vi "DAC Configure FP View.vi"(8 "error in":errorcluster, 11 "DAC RTD Temp in":refnum<class "DAC RTD Temp.lvclass">) -> (0 "error out":errorcluster, 3 "DAC RTD Temp out":refnum<class "DAC RTD Temp.lvclass">)   [LabVIEW 2019, in "DAC.lvlib" / "DAC RTD Temp.lvclass"]
uses:
  DAC RTD Temp.lvclass
  DAC RTD Temp.lvclass/DAC RTD Temp.ctl
  Results/Heat Flow Results/Heat Flow Results.lvclass/Heat Flow Results.ctl
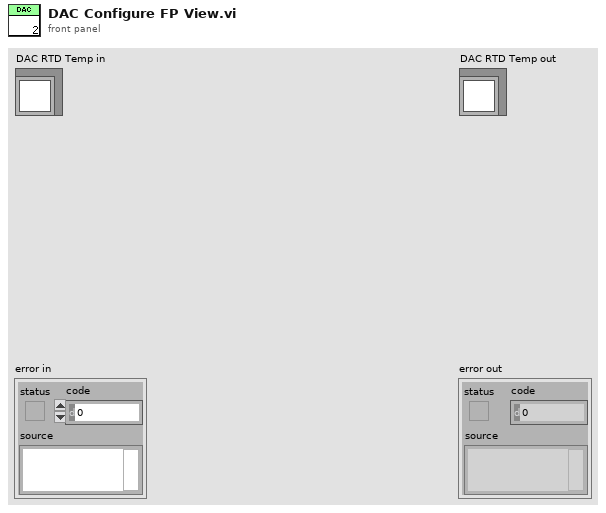
[diagram p1: front panel]
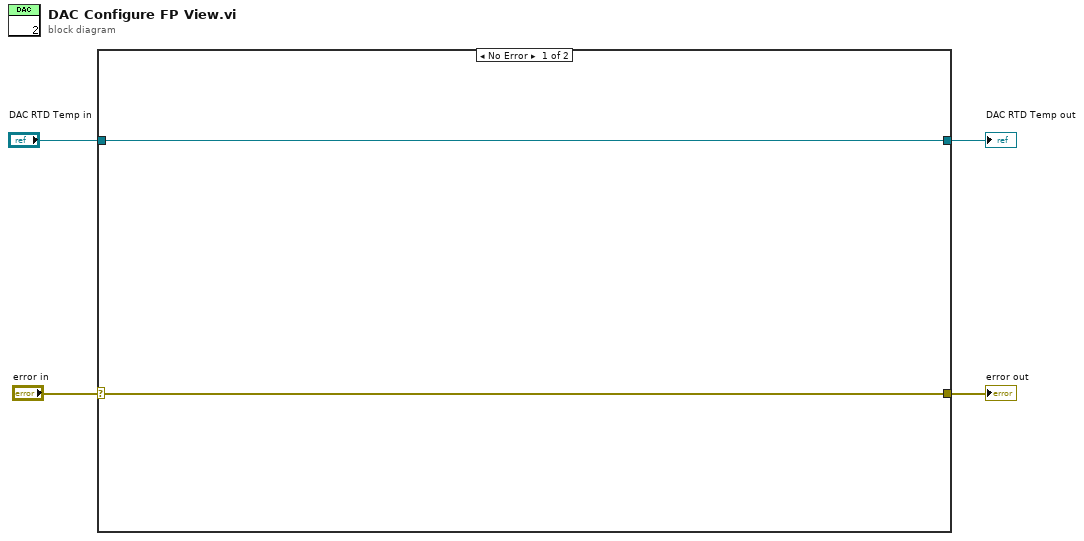
[diagram p0: block diagram]
diagram:
  n1 = case shown="No Error" "error in" {
    selector: "error in" -> [w5 w8]
    tunnel: [w5 w8] -> w1
    tunnel: [w6 w7] -> w2
    tunnel: "DAC RTD Temp in" -> [w6 w7]
    frame No Error {
    }
    frame Error {
    }
  }
  "error out" <- w1
  "DAC RTD Temp out" <- w2
